vi "TektronixMDO_singleChannelReadout_writeFile.vi"() -> ()   [LabVIEW 2016]
doc: "This example illustrates how to use autosetup and continuously acquires waveforms from a single channel using the following steps:\n\n1. Specify a valid VISA session. \n2. Specify a channel. \n3. Specify a time-out value for reading waveform.\n4. Run the VI. The graph displays the waveform you acquire."
uses:
  <instrlib>/Tektronix DPO MSO 2000 4000 Series/Public/Configure/Configure Trigger (Edge).vi
  <instrlib>/Tektronix DPO MSO 2000 4000 Series/Public/Data/Read (Single Waveform).vi
  <instrlib>/Tektronix DPO MSO 2000 4000 Series/Tektronix DPO MSO 2000 4000 Series.lvlib
panel:
  out "Event rate":dbl
  in  "Maximum Time (10000ms)":u32=10000
  in  "Probe Attenuation (1)":dbl=1.0
  in  "Bandwidth (0: FULL)":u16(ring) items=["FULL", "250 MHz", "150 MHz", "20 MHz"]
  in  "Vertical Offset (0.0 V)":dbl
  in  "Vertical Range (10.0 V)":dbl=10.0
  in  "Vertical Coupling (1: DC)":u16(ring)=1 items=["AC", "DC", "Ground", "DC Reject"]
  in  "Input Impedance (0: 1M ohm)":u16(ring) items=["1M", "75", "50"]
  out "Event Count":i32
  in  "Target total event":i32
  out "dt":dbl format="%#_13g"
  out "Histogram":dynamicdata(graph)
  in  "Operator":string="Hsin-Yeh"
  in  "file path":path=path "C:/Users/NTU/Desktop/Chih-Ping/NaI0827/1-haveNumber/Co60/Co60_5.tdms"
  in  "Timebase (0.0005 s)":dbl=0.0005
  in  "Position (10 %)":dbl=10.0
  in  "Record Length (10: 10k points)":u32(ring)=10 items=["1000 points"=1, "10k points"=10, "100k points"=100, "1M points"=1000, "5M points"=5000, "10M points"=10000]
  in  "Trigger Slope (0: Rising)":u16(ring) items=["Rising", "Falling", "Either"]
  in  "Trigger Level (0.0 V)":dbl
  in  "Trigger Coupling (0 : DC)":u16(ring) items=["DC", "HF Reject", "LF Reject", "Noise Reject", "AC"]
  in  "Channel (0: Channel 1)":u16(ring) items=["Channel 1", "Channel 2", "Channel 3", "Channel 4", "Math", "Reference 1", "Reference 2", "Reference 3", "Reference 4"]
  out "Waveform Graph":waveform(dbl)(graph)
  in  "Enable Channel (T: Enable)":bool=TRUE
  in  "stop":bool
  in  "VISA Resource Name":refnum<visa-resource-name>
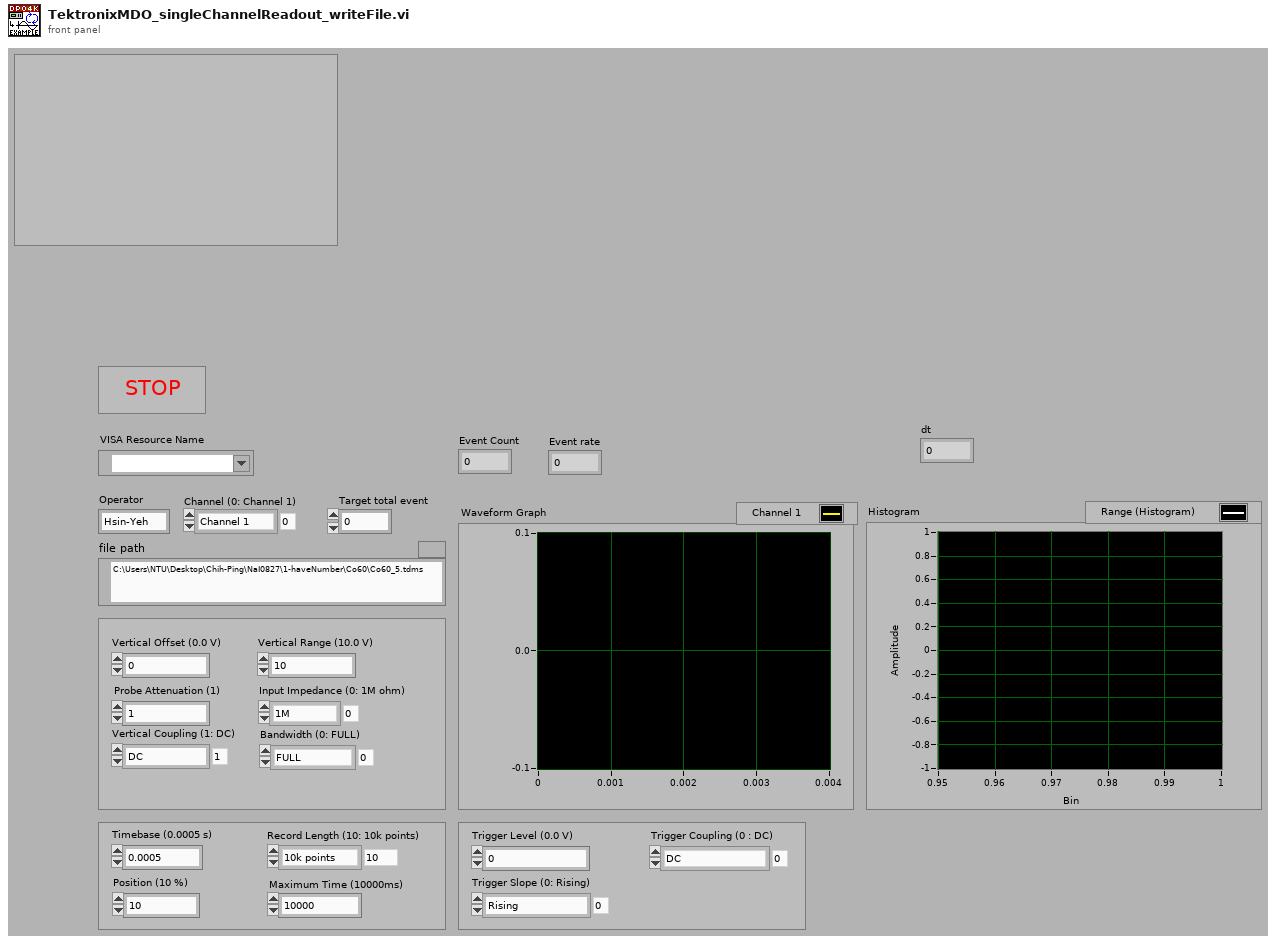
[diagram p1: front panel]
types:
  T1 = enum16{"open", "open or create", "create or replace", "create", "open (read-only)"}
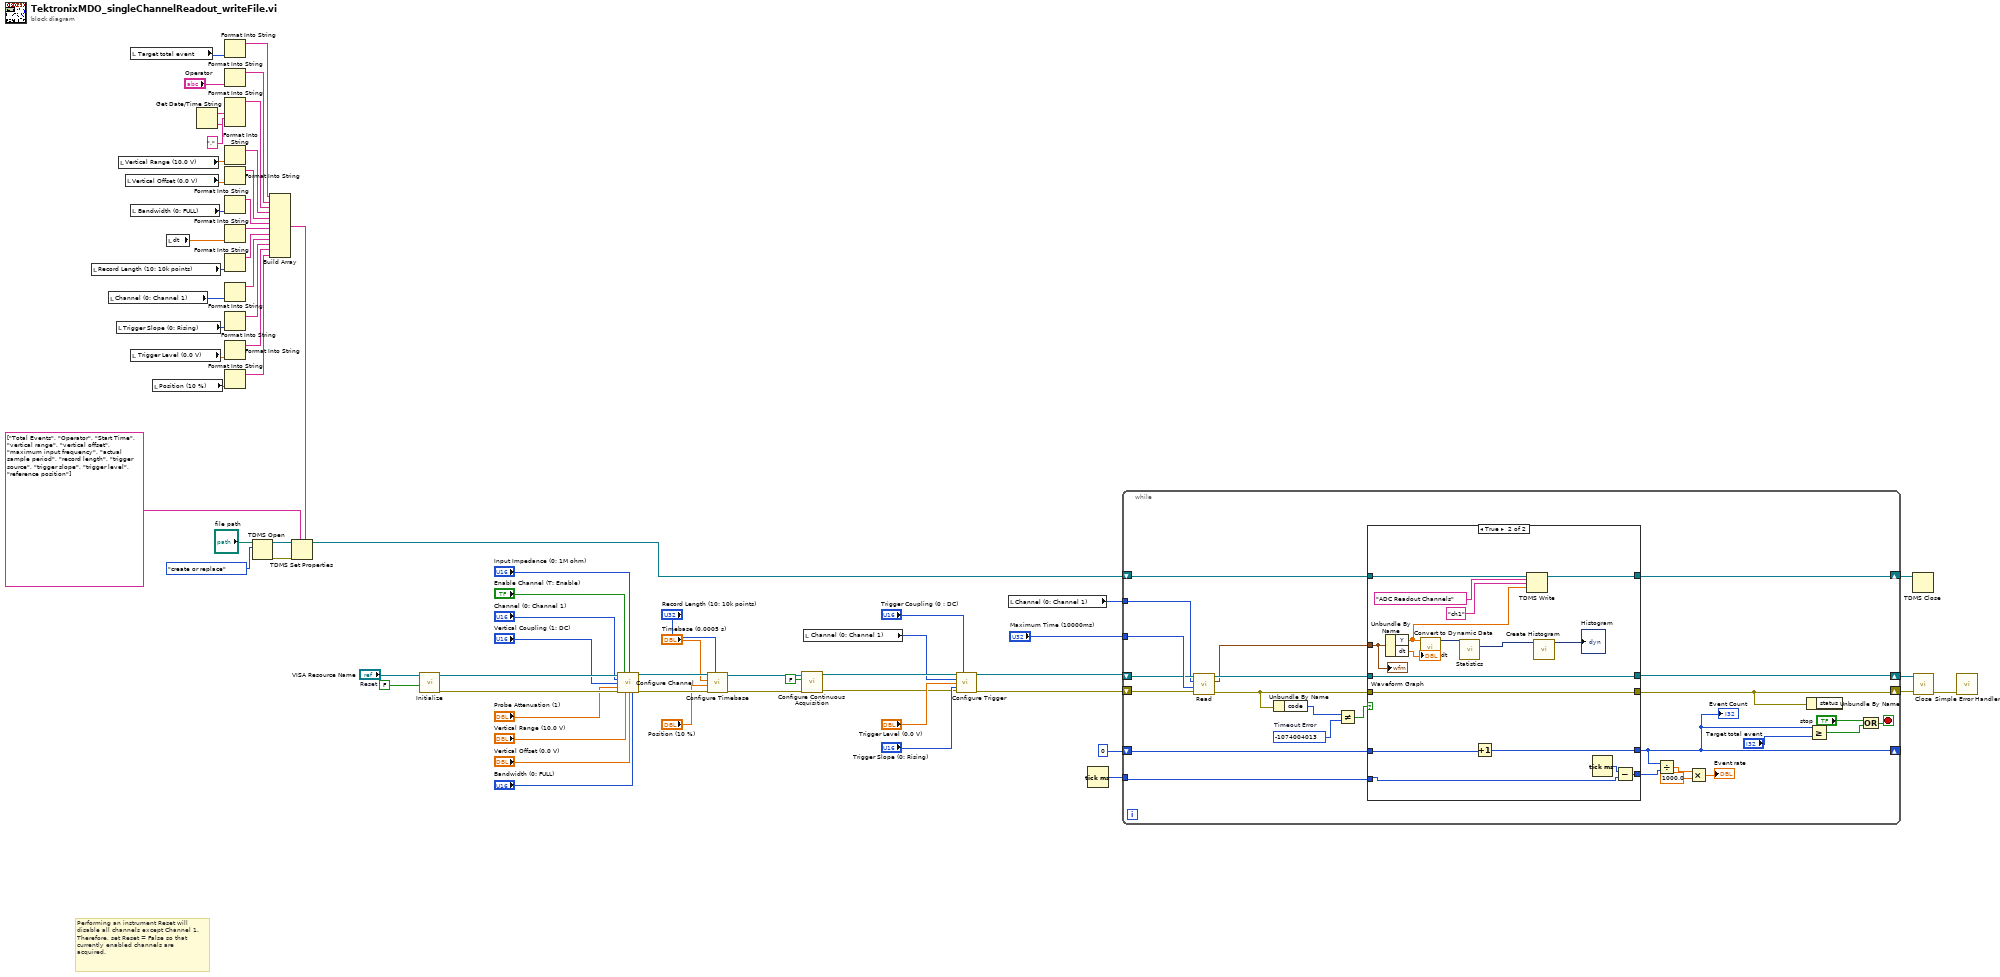
[diagram p0: block diagram]
diagram:
  w66 = FALSE  # Reset
  # "Performing an instrument Reset will disable all channels except Channel 1. Therefore, set Reset = False so that currently enabled channels are acquired."
  n1 = local read "Record Length (10: 10k points)"() -> (w41:u32)
  n2 = local read "Channel (0: Channel 1)"() -> (w40:u16)
  n3 = local read "Trigger Slope (0: Rising)"() -> (w27:u16)
  n4 = local read "Vertical Range (10.0 V)"() -> (w39:dbl)
  n5 = local read "Vertical Offset (0.0 V)"() -> (w36:dbl)
  n6 = local read "Target total event"() -> (w15:i32)
  n7 = local read "Bandwidth (0: FULL)"() -> (w35:u16)
  n8 = local read "Trigger Level (0.0 V)"() -> (w42:dbl)
  n9 = local read "Position (10 %)"() -> (w37:dbl)
  n10 = local read "dt"() -> (w38:dbl)
  n11 = Get Date/Time String() -> (date string=w33:string, time string=w31:string)  [unwired: 3 in]
  n12 = Format Into String(w15) -> (resulting string=w43:string)  [unwired: 3 in, 1 out]
  n13 = Format Into String("Operator") -> (resulting string=w30:string)  [unwired: 3 in, 1 out]
  n14 = Format Into String(w33, "," ("input 2"), w31) -> (resulting string=w29:string)  [unwired: 3 in, 1 out]
  n15 = Format Into String(w39) -> (resulting string=w28:string)  [unwired: 3 in, 1 out]
  n16 = Format Into String(w36) -> (resulting string=w25:string)  [unwired: 3 in, 1 out]
  n17 = Format Into String(w35) -> (resulting string=w26:string)  [unwired: 3 in, 1 out]
  n18 = Format Into String(w38) -> (resulting string=w24:string)  [unwired: 3 in, 1 out]
  n19 = Format Into String(w41) -> (resulting string=w23:string)  [unwired: 3 in, 1 out]
  n20 = Format Into String(w40) -> (resulting string=w22:string)  [unwired: 3 in, 1 out]
  n21 = Format Into String(w27) -> (resulting string=w21:string)  [unwired: 3 in, 1 out]
  n22 = Format Into String(w42) -> (resulting string=w20:string)  [unwired: 3 in, 1 out]
  n23 = Format Into String(w37) -> (resulting string=w19:string)  [unwired: 3 in, 1 out]
  n24 = TDMS Open(10:T1."create or replace" ("operation (0:open)"), 11:"file path") -> (0:w45:errorcluster, 3:w44:refnum<k34>)  [unwired: 5 in]
  n25 = Build Array(w43, w30, w29, w28, w25, w26, w24, w23, w22, w21, w20, w19) -> (w18:string[])
  n26 = TDMS Set Properties(5:w18, 7:string[] ["Total Events", "Operator", "Start Time", "vertical range", "vertical offset", "maximum input frequency", "actual sample period", "record length", "trigger source", "trigger slope", "trigger level", "reference position"], 8:w45, 11:w44) -> (3:w14:refnum<k34>)  [unwired: 2 in, 3 out]
  n27 = call <instrlib>:"Initialize.vi"("Reset (True)"=w66, "VISA resource name"="VISA Resource Name") -> ("error out"=w63:errorcluster, "VISA resource name out"=w64:refnum<visa-resource-name>)  [unwired: 8 in]
  n28 = call <instrlib>:"Configure Channel.vi"("VISA resource name"=w64, "Enable Channel (T: Enable)"="Enable Channel (T: Enable)", "Input Impedance (0: 1M ohm)"="Input Impedance (0: 1M ohm)", "Channel (0: Channel 1)"="Channel (0: Channel 1)", "Vertical Coupling (1: DC)"="Vertical Coupling (1: DC)", "Probe Attenuation (1)"="Probe Attenuation (1)", "error in (no error)"=w63, "Vertical Range (10.0 V)"="Vertical Range (10.0 V)", "Vertical Offset (0.0 V)"="Vertical Offset (0.0 V)", "Bandwidth (0: FULL)"="Bandwidth (0: FULL)") -> ("VISA resource name out"=w52:refnum<visa-resource-name>, "error out"=w51:errorcluster)  [unwired: 4 in]
  n29 = call <instrlib>:"Configure Timebase.vi"("Record Length (10: 10k points)"="Record Length (10: 10k points)", "error in (no error)"=w51, "Position (10 %)"="Position (10 %)", "Timebase (0.0005 s)"="Timebase (0.0005 s)", "VISA resource name"=w52) -> ("error out"=w7:errorcluster, "VISA resource name out"=w9:refnum<visa-resource-name>)  [unwired: 5 in]
  n30 = call <instrlib>:"Configure Continuous Acquisition.vi"("error in (no error)"=w7, "Enable Continuous Acquisition Mode (T: Enable)"=FALSE, "VISA resource name"=w9) -> ("error out"=w6:errorcluster, "VISA resource name out"=w8:refnum<visa-resource-name>)  [unwired: 7 in]
  n31 = local read "Channel (0: Channel 1)"() -> (w2:u16)
  n32 = call-poly <instrlib>:"Configure Trigger.vi"("VISA resource name"=w8, "Trigger Coupling (0 : DC)"="Trigger Coupling (0 : DC)", "Trigger Source (0: Channel 1)"=w2, "Trigger Level (0.0 V)"="Trigger Level (0.0 V)", "Trigger Slope (0: Rising)"="Trigger Slope (0: Rising)", "error in (no error)"=w6) -> ("VISA resource name out"=w17:refnum<visa-resource-name>, "error out"=w11:errorcluster)  [unwired: 8 in]
  n33 = local read "Channel (0: Channel 1)"() -> (w3:u16)
  n34 = Tick Count (ms)() -> (millisecond timer value=w1:u32)
  n35 = while {
    tunnel: "Maximum Time (10000ms)" -> [w93]
    shift-right: [w90] -> w68
    shift-left: w17 -> [w92]
    shift-right: [w80] -> w12
    shift-left: w14 -> [w81]
    shift-right: [w74] -> _
    shift-left: 0 -> [w86]
    shift-right: [w78] -> w10
    shift-left: w11 -> [w79]
    tunnel: w3 -> [w76]
    tunnel: w1 -> [w75]
    stop <- w82 stop-if-true
    w88 = -1074004013  # Timeout Error
    n36 = call-poly <instrlib>:"Read.vi"("error in (no error)"=w79, "Maximum Time (10000ms)"=w93, "Channel (0: Channel 1)"=w76, "VISA resource name"=w92) -> ("error out"=w78:errorcluster, "Waveform Graph"=w77:waveform(dbl), "VISA resource name out"=w91:refnum<visa-resource-name>)  [unwired: 5 in]
    n37 = Unbundle By Name(w78) -> ("code"=w89:i32)
    n38 = Not Equal?(x=w89, y=w88) -> (x != y?=w87:bool)
    n39 = case shown="True" w87 {
      tunnel: w91 -> [w98 w109]
      tunnel: [w98 w109] -> w90
      tunnel: w78 -> [w97 w105]
      tunnel: [w97 w105] -> _
      tunnel: w86 -> [w96 w114]
      tunnel: [w96 w113] -> w74
      tunnel: w81 -> [w95 w112]
      tunnel: [w95 w110] -> w80
      tunnel: w77 -> [_ w104]
      tunnel: w75 -> [w94 w100]
      tunnel: [w94 w99] -> w73
      frame False {
      }
      frame True {
        n40 = Unbundle By Name(w104) -> ("Y"=w107:dbl[], "dt"=→"dt":dbl)
        n41 = call "Convert to Dynamic Data"("Array"=w107) -> ("Dynamic Data Type"=w108:dynamicdata)  [unwired: 3 in]
        n42 = call "Statistics"("Signals"=w108) -> ("Range"=w103:dynamicdata)  [unwired: 25 in, 1 out]
        n43 = Increment(x=w114) -> (x+1=w113:i32)
        n44 = TDMS Write(0:w112, 5:"ADC Readout Channels" ("group name (Untitled)"), 7:"ch1", 9:w107) -> (4:w110:refnum<k34>)  [unwired: 2 in, 3 out]
        n45 = call "Create Histogram"("Signal"=w103) -> ("Histogram"=→"Histogram":dynamicdata)  [unwired: 9 in, 1 out]
        n46 = Tick Count (ms)() -> (millisecond timer value=w101:u32)
        n47 = Subtract(x=w101, y=w100) -> (x-y=w99:u32)
        "Waveform Graph" <- w104
      }
    }
    "Event Count" <- w74
    n48 = Divide(x=w74, y=w73) -> (x/y=w72:dbl)
    n49 = Multiply(x=w72, y=1000.0) -> (x*y=→"Event rate":dbl)
    n50 = Unbundle By Name(w78) -> ()  [unwired: 1 out]
    n51 = Greater Or Equal?(x=w74, y="Target total event") -> (x >= y?=w83:bool)
    n52 = Compound Arithmetic op=OR("stop", w83) -> (w82:bool)
  }
  n53 = TDMS Close(11:w12) -> ()  [unwired: 1 in, 2 out]
  n54 = call <instrlib>:"Close.vi"("error in (no error)"=w10, "VISA resource name"=w68) -> ("error out"=w67:errorcluster)  [unwired: 9 in]
  n55 = call <vilib>:"Simple Error Handler.vi"("error in (no error)"=w67) -> ()  [unwired: 4 in, 5 out]
